vi "Write to Log Buffer.vi"(1 "error in":errorcluster, 2 "array of values":dbl[](array[numeric])=[0.0, 0.0, 0.0, 0.0, 0.0, 0.0, 0.0]) -> (0 "error out":errorcluster)   [LabVIEW 2016]
uses:
  Refname/Queues.ctl
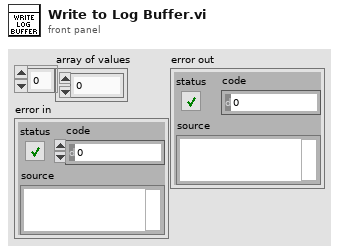
[diagram p1: front panel]
types:
  T1 = typedef "Queues.ctl" = enum16{"Log Queue"}
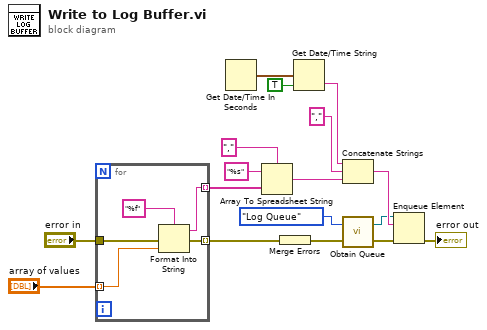
[diagram p0: block diagram]
diagram:
  n1 = for {
    tunnel: "array of values" -> [w22] mode=indexing
    tunnel: [w20] -> w15 mode=indexing
    tunnel: "error in" -> [w19]
    tunnel: [w18] -> w6 mode=indexing
    n2 = Format Into String(format string="%f", error in=w19, w22) -> (resulting string=w20:string, error out=w18:errorcluster)  [unwired: 1 in]
  }
  n3 = Get Date/Time In Seconds() -> (seconds since 1Jan1904=w14:timestamp)
  n4 = Array To Spreadsheet String(delimiter (Tab)=",", array=w15, 3:"%s" ("format string")) -> (spreadsheet string=w10:string)
  n5 = Merge Errors(w6) -> (w2:errorcluster)
  n6 = Get Date/Time String(seconds (now)=w14, want seconds? (F)=TRUE) -> (time string=w12:string)  [unwired: 1 in, 1 out]
  n7 = Concatenate Strings(w12, "," ("string"), w10) -> (w8:string)
  n8 = call "Obtain Queue.vi"("error in"=w2, "Queue"=Queues."Log Queue") -> ("error out"=w3:errorcluster, "Queue Ref"=w4:refnum<queue>)
  n9 = Enqueue Element(queue=w4, element=w8, error in (no error)=w3) -> (error out=→"error out":errorcluster)  [unwired: 1 in, 2 out]
